vi "peak - less simple guess at omega.vi"(10 "omega":dbl[](array[numeric]), 11 "Unwrapped Phase":dbl[](array[numeric])) -> (2 "gamma guess":dbl, 3 "omega guess":dbl)   [LabVIEW 2017]
uses:
  <vilib>/gmath/NI_Gmath.lvlib
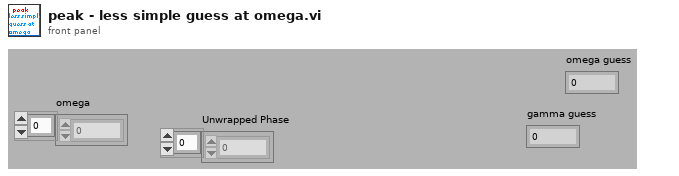
[diagram p1: front panel]
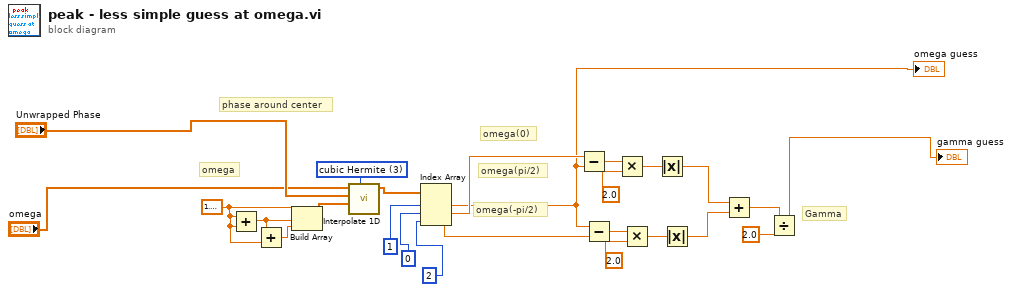
[diagram p0: block diagram]
diagram:
  w11 = 1.5707963267948966
  w13 = 3 items=["nearest", "linear", "spline", "cubic Hermite", "Lagrange"] ("method")
  # "phase around center"
  # "omega"
  # "omega(-pi/2)"
  # "omega(pi/2)"
  # "omega(0)"
  # "Gamma"
  n1 = Add(x=w11, y=w11) -> (x+y=w12:dbl)
  n2 = Add(x=w12, y=w11) -> (x+y=w10:dbl)
  n3 = Build Array(w11, w12, w10) -> (w9:dbl[])
  n4 = call <vilib>:"Interpolate 1D.vi"("method"=w13, "xi"=w9, "X"="Unwrapped Phase", "Y"="omega") -> ("yi"=w5:dbl[])  [unwired: 5 in, 2 out]
  n5 = Index Array(array=w5, index #1=1, index #2=0, index #3=2) -> (element #1=w1:dbl, element #2=w4:dbl, element #3=w3:dbl)
  "omega guess" <- w1
  n6 = Subtract(x=w4, y=w1) -> (x-y=w23:dbl)
  n7 = Subtract(x=w1, y=w3) -> (x-y=w20:dbl)
  n8 = Multiply(x=w23, y=2.0) -> (x*y=w21:dbl)
  n9 = Multiply(x=w20, y=2.0) -> (x*y=w18:dbl)
  n10 = Absolute Value(x=w21) -> (abs(x)=w17:dbl)
  n11 = Absolute Value(x=w18) -> (abs(x)=w14:dbl)
  n12 = Add(x=w17, y=w14) -> (x+y=w16:dbl)
  n13 = Divide(x=w16, y=2.0) -> (x/y=→"gamma guess":dbl)
